vi "Add To Scan Log.vi"(0 "Model in":refnum<class "Model.lvclass">, 5 "Control Value":dbl, 7 "Measured Force":dbl[unit], 11 "error in (no error)":errorcluster) -> (4 "Model out":refnum<class "Model.lvclass">, 15 "error out":errorcluster)   [LabVIEW 2015]
uses:
  Model.lvclass
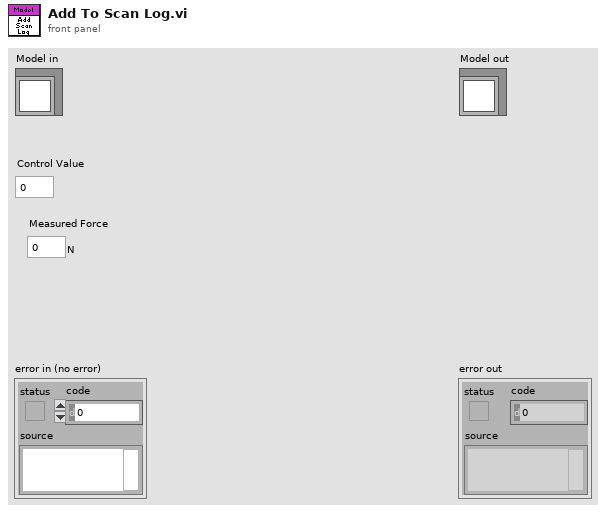
[diagram p1: front panel]
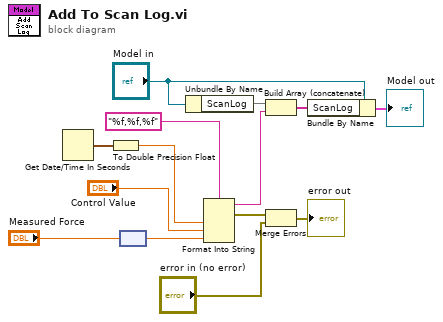
[diagram p0: block diagram]
diagram:
  n1 = Get Date/Time In Seconds() -> (seconds since 1Jan1904=w3:timestamp)
  n2 = To Double Precision Float(number=w3) -> (double precision float=w2:dbl)
  n3 = node("Measured Force") -> (w4:dbl)
  n4 = Unbundle By Name("Model in") -> ("ScanLog"=w14)
  n5 = Format Into String(format string="%f,%f,%f", w2, "Control Value", w4) -> (resulting string=w10:string, error out=w8:errorcluster)  [unwired: 2 in]
  n6 = Build Array (concatenate)(w14, w10) -> (w9:string[])
  n7 = Merge Errors(w8, "error in (no error)") -> (→"error out":errorcluster)
  n8 = Bundle By Name(cluster="Model in", "ScanLog"=w9) -> (→"Model out":cluster{})
